vi "Set Plugin Enabled.vi"(8 "error in (no error)":errorcluster, 9 "Enabled?":bool, 10 "Plugin":string) -> (0 "error out":errorcluster)   [LabVIEW 2020, in "UI Configuration Manager.lvclass"]
uses:
  UI Configuration Manager.lvclass
  Framework/Configuration Manager/Configuration Manager.lvclass
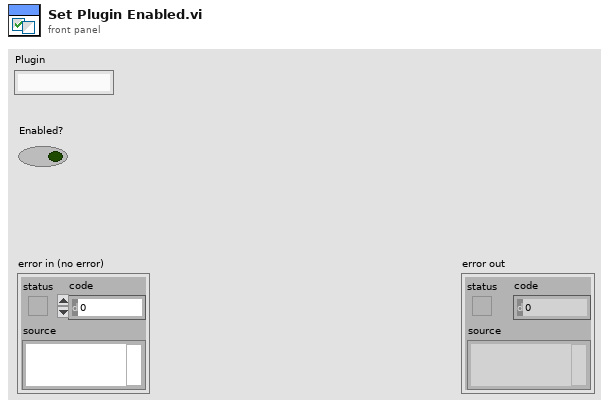
[diagram p1: front panel]
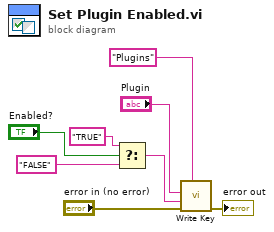
[diagram p0: block diagram]
diagram:
  n1 = Select(t="TRUE" ("key"), s="Enabled?", f="FALSE") -> (s? t:f=w1:string)
  n2 = call "Write Key.vi"("section"="Plugins", "error in (no error)"="error in (no error)", "value"=w1, "key"="Plugin") -> ("error out"=→"error out":errorcluster)  [unwired: 7 in]
